vi "Load Hardware.vi"(8 "error in (no error)":errorcluster, 10 "Program only changes":bool=TRUE, 11 "Arduino DDS in":refnum<class "Arduino DDS.lvclass">) -> (0 "error out":errorcluster, 3 "Arduino DDS out":refnum<class "Arduino DDS.lvclass">)   [LabVIEW 2013, in "Arduino DDS.lvclass"]
uses:
  Arduino DDS.lvclass
  Device/Device.lvclass
panel:
  # "encapsulate HWI in cluser so each \"last encountered\"\ncan be a different length."
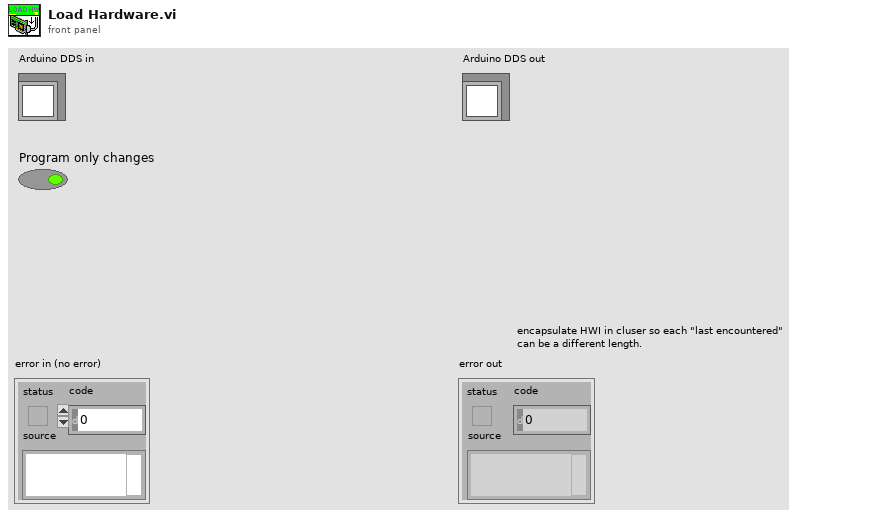
[diagram p1: front panel]
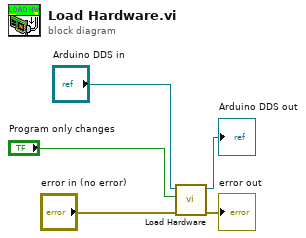
[diagram p0: block diagram]
diagram:
  n1 = call-parent "Load Hardware.vi"("error in (no error)"="error in (no error)", "Program only changes"="Program only changes", "Device in"="Arduino DDS in") -> ("error out"=→"error out":errorcluster, "Device out"=→"Arduino DDS out":refnum<class "Arduino DDS.lvclass">)  [unwired: 7 in]
